vi "WinCI Get Project Path.vi"(8 "error in (no error)":errorcluster, 9 "configuration data in":string, 11 "source control reference in":T1) -> (0 "error out":errorcluster, 1 "configuration data out":string, 2 "status message":string, 3 "source control reference out":T1, 5 "dialog box cancelled?":bool)   [LabVIEW 2020, in "NI_SCC_WinCI.lvlib"]
uses:
  <vilib>/SourceControl/Providers/WinCI/NI_SCC_WinCI.lvlib
  <vilib>/SourceControl/sccapi/SCCAPI Refnum.ctl
  <vilib>/SourceControl/support/SCCSup ConfigData Conv.ctl
  <vilib>/SourceControl/Providers/WinCI/WinCI SCC Project Details.ctl
  <vilib>/SourceControl/support/SCCSup Message Strings GLBL.vi
  <vilib>/SourceControl/sccapi/NI_SCC.lvlib
panel:
  out "result":i32
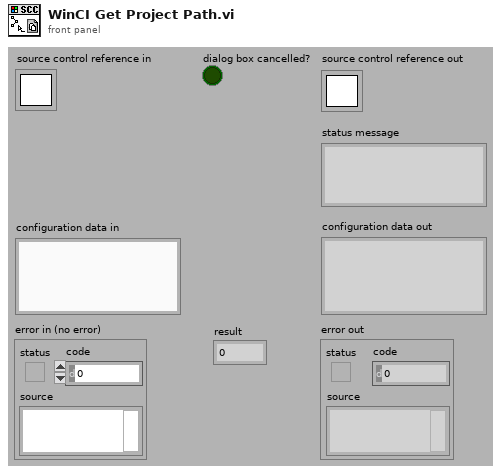
[diagram p1: front panel]
types:
  T1 = typedef "NI_SCC.lvlib/SCCAPI Refnum.ctl" = refnum<k1>
  T2 = typedef "SCCSup ConfigData Conv.ctl" = enum16{"from config data", "to config data"}
  T3 = typedef "NI_SCC_WinCI.lvlib/WinCI SCC Project Details.ctl" = cluster{"user name":string, "project name":string, "local path":string, "database name":string}
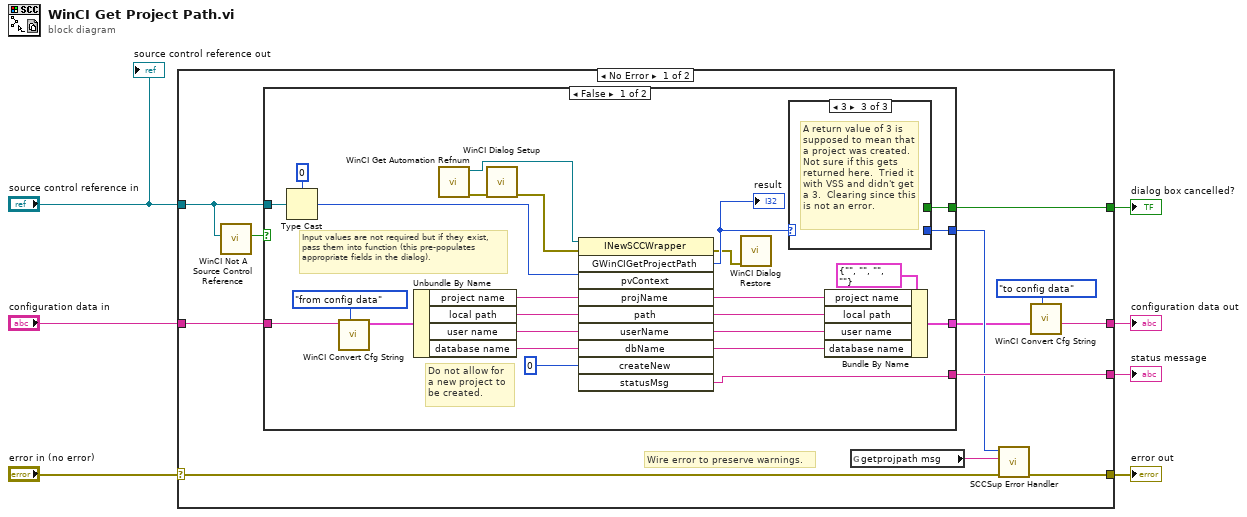
[diagram p0: block diagram]
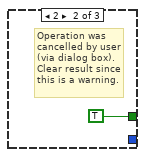
[diagram p3: hidden frame]
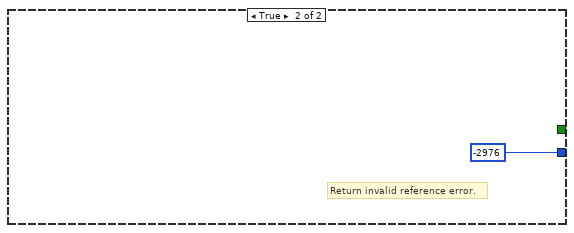
[diagram p4: hidden frame]
diagram:
  n1 = case shown="No Error" "error in (no error)" {
    selector: "error in (no error)" -> [w15 w48]
    tunnel: [w19 w48] -> w6
    tunnel: [w18 _] -> w5
    tunnel: "source control reference in" -> [w8 _]
    tunnel: [w14 _] -> w3
    tunnel: [w11 _] -> w2
    tunnel: "configuration data in" -> [w13 _]
    frame No Error {
      # "Wire error to preserve warnings."
      n2 = call <vilib>:"WinCI Not A Source Control Reference.vi"("source control reference in"=w8) -> ("not a source control reference?"=w9:bool)  [unwired: 1 in, 9 out]
      n3 = case shown="False" w9 {
        tunnel: [w44 _] -> w12
        tunnel: [w30 _] -> w18
        tunnel: [w41 -2976 ("result")] -> w17
        tunnel: w8 -> [w42 _]
        tunnel: [w40 _] -> w14
        tunnel: w13 -> [w37 _]
        frame False {
          # "Input values are not required but if they exist, pass them into function (this pre-populates appropriate fields in the dialog)."
          # "Do not allow for a new project to be created."
          n4 = Type Cast(type=u32 0, x=w42) -> (*(type *) &x=w35:u32)
          n5 = call <vilib>:"WinCI Convert Cfg String.vi"("conversion action"=SCCSup_ConfigData_Conv."from config data", "config data in"=w37) -> ("project details out"=w36:T3)  [unwired: 1 in, 8 out]
          n6 = Unbundle By Name(w36) -> ("project name"=w34:string, "local path"=w33:string, "user name"=w32:string, "database name"=w31:string)
          n7 = call <vilib>:"WinCI Get Automation Refnum.vi"() -> ("error out"=w22:errorcluster, "automation refnum"=w25:refnum<k7>)  [unwired: 10 out]
          n8 = call <vilib>:"WinCI Dialog Setup.vi"("error in"=w22) -> ("error out"=w21:errorcluster)  [unwired: 10 out]
          n9 = invoke class="INewSCCWrapper" method="GWinCIGetProjectPath"(reference=w25, error in=w21, "pvContext"=w35, "projName"=w34, "path"=w33, "userName"=w32, "dbName"=w31, "createNew"=0) -> (error out=w20:errorcluster, "GWinCIGetProjectPath"=w23:i32, "projName"=w29:string, "path"=w28:string, "userName"=w27:string, "dbName"=w26:string, "statusMsg"=w30:string)  [unwired: 2 in, 3 out]
          "result" <- w23
          n10 = call <vilib>:"WinCI Dialog Restore.vi"("error in"=w20) -> ()  [unwired: 11 out]
          n11 = case shown="3" w23 {
            selector: w23 -> [w45 _ _]
            tunnel: [w45 _ _] -> w41
            tunnel: [_ TRUE _] -> w40
            frame Default {
            }
            frame 2 {
              # "Operation was cancelled by user (via dialog box).  Clear result since this is a warning."
            }
            frame 3 {
              # "A return value of 3 is supposed to mean that a project was created.  Not sure if this gets returned here.  Tried it with VSS and didn't get a 3.  Clearing since this is not an error."
            }
          }
          n12 = Bundle By Name(cluster=T3 {"user name"="", "project name"="", "local path"="", "database name"=""} ("returned project details"), "project name"=w29, "local path"=w28, "user name"=w27, "database name"=w26) -> (w44:T3)
        }
        frame True {
          # "Return invalid reference error."
        }
      }
      n13 = global read "SCCSup Message Strings GLBL.vi" "getprojpath msg"() -> (w16:string)
      n14 = call <vilib>:"SCCSup Error Handler.vi"("error in (no error)"=w15, "operation message"=w16, "scc error code"=w17) -> ("error out"=w19:errorcluster)  [unwired: 1 in, 7 out]
      n15 = call <vilib>:"WinCI Convert Cfg String.vi"("conversion action"=SCCSup_ConfigData_Conv."to config data", "project details in"=w12) -> ("config data out"=w11:string)  [unwired: 1 in, 8 out]
    }
    frame Error {
    }
  }
  "error out" <- w6
  "status message" <- w5
  "dialog box cancelled?" <- w3
  "configuration data out" <- w2
  "source control reference out" <- "source control reference in"
